vi "Get grpc-library ref.vi"(8 "error in":errorcluster) -> (0 "error out":errorcluster, 3 "Library out":refnum<vi>)   [LabVIEW 2019, in "gRPC Template Creation Utility.lvlib"]
uses:
  gRPC Template Creation Utility.lvlib
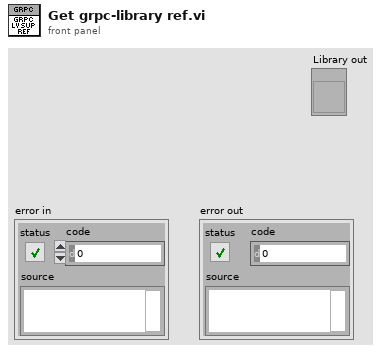
[diagram p1: front panel]
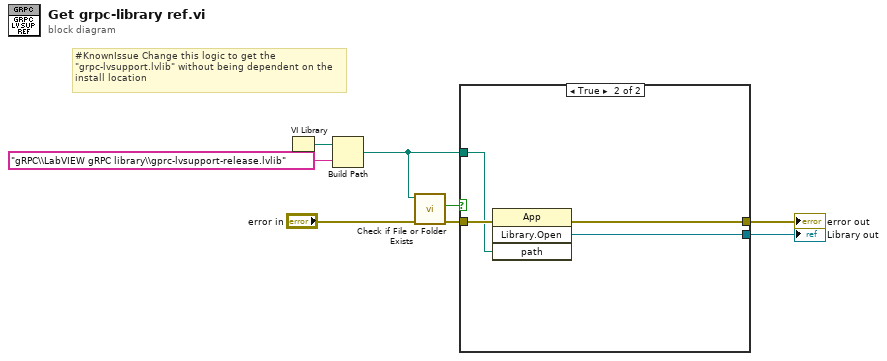
[diagram p0: block diagram]
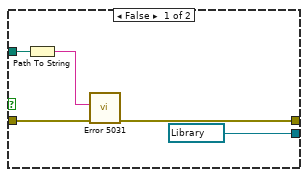
[diagram p2: hidden frame]
diagram:
  # "#KnownIssue Change this logic to get the \"grpc-lvsupport.lvlib\" without being dependent on the install location"
  n1 = VI Library() -> (path=w8:path)
  n2 = Build Path(base path=w8, name or relative path="gRPC\\LabVIEW gRPC library\\gprc-lvsupport-release.lvlib") -> (appended path=w2:path)
  n3 = call <vilib>:"Check if File or Folder Exists.vi"("error in (no error)"="error in", "path"=w2) -> ("error out"=w3:errorcluster, "file or folder exists?"=w1:bool)  [unwired: 7 in, 1 out]
  n4 = case shown="True" w1 {
    tunnel: [refnum<vi> refnum ("Open Library") w17] -> w6
    tunnel: [w11 w16] -> w5
    tunnel: w3 -> [w12 w15]
    tunnel: w2 -> [w10 w14]
    frame False {
      n5 = Path To String(path=w10) -> (string=w9:string)
      n6 = call "Error 5031.vi"("error in (no error)"=w12, "Location"=w9) -> ("error out"=w11:errorcluster)  [unwired: 9 in]
    }
    frame True {
      n7 = invoke class="App" method="Library.Open"(error in=w15, "path"=w14) -> (error out=w16:errorcluster, "Open Library"=w17:refnum<vi>)  [unwired: 2 in, 2 out]
    }
  }
  "error out" <- w5
  "Library out" <- w6
